vi "UART_Firmware_MultiUp.vi"() -> ()   [LabVIEW 2012]
uses:
  <vilib>/Platform/TimedLoop/XDataNode/timing_clust.ctl
  <vilib>/Platform/TimedLoop/XDataNode/nitl_modes.ctl
  <vilib>/Platform/TimedLoop/XDataNode/wakeup.ctl
  UART/UART_Command.ctl
  <vilib>/rvi/eio/common/nirviEmuTemplateMethod_errors.vi
  <vilib>/rvi/Emulation/niFpgaSctlEmulationRegisterWithScheduler.vi
  <vilib>/rvi/Emulation/niFpgaSctlEmulationScheduler.vi
  <vilib>/eio/EIONode/EIONode.xnode
  <vilib>/Platform/TimedLoop/XDataNode/XDataNode.xnode
  UART/UART_Firmware.lvlib
  <vilib>/Platform/TimedLoop/XDataNode/XDNodeRunTimeDep.lvlib
panel:
  out "FPGA Initialization Complete?":bool
  out "Maximum Nup?":u8
  out "Rx1 FIFO T.O.?":bool
  out "Rx FIFO T.O.?":bool
  out "Tx FIFO T.O.?":bool
  out "Rx0 FIFO T.O.?":bool
  out "IO Module Pre Setup Complete?":bool
  out "Set Voltage Done":bool
  in  "Voltage_Family":u8=4
  out "IO Enabled":bool
  out "DCM_Locked":bool
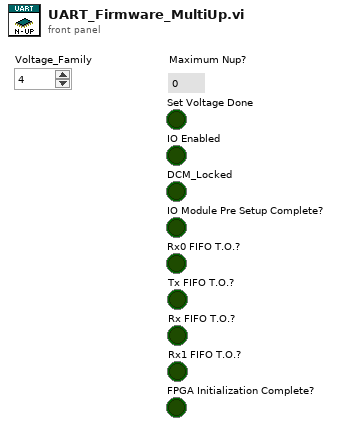
[diagram p1: front panel]
types:
  T1 = typedef "UART_Firmware.lvlib/UART_Command.ctl" = enum8{"None", "Tx", "SetBaud_High", "SetBaud_Low", "SetCharLength", "SetParity", "SetStopBits", "SetSpacing_High", "SetSpacing_Low"}
  T2 = typedef "XDNodeRunTimeDep.lvlib/timing_clust.ctl" = cluster{"Expected End [f-1]":u64, "Actual End [f-1]":u64, "Finished Late? [f-1]":bool, "Expected End [i-1]":u64, "Actual End [i-1]":u64, "Finished Late? [i-1]":bool, "Expected Start [i]":u64, "Actual Start [i]":u64, "Expected Start [f]":u64, "Actual Start [f]":u64, "Source Name":string, "Structure Name":string, "Period":i64, "Deadline":i64, "Offset":i64, "Start":i64, "Priority":i32, "Timeout":i32, "Mode":T3, "Wakeup Reason":T4, "Error":errorcluster, "Source Type":string, "Secondary Source Type":string, "Global End Time":u64, "Global Start Time":u64, "Frame Duration":u64, "Iteration Duration":u64, "Assigned CPU":i32, "I/O Scan Engine Mode":u32}
  T3 = typedef "XDNodeRunTimeDep.lvlib/nitl_modes.ctl" = enum32{"No Change", "Process missed periods, maintain original phase", "Discard missed periods, maintain original phase", "Process missed periods, ignore original phase", "Discard missed periods, ignore original phase"}
  T4 = typedef "XDNodeRunTimeDep.lvlib/wakeup.ctl" = enum32{"Normal", "Aborted", "Asynchronous wakeup", "Timing source error", "Timed loop error", "Timeout"}
  T5 = typedef "UART_Firmware.lvlib/UART_Response.ctl" = enum8{"None", "Rx", "BaudHighAck", "BaudLowAck", "CharSizeAck", "ParityAck", "StopBitsAck", "SpacingHighAck", "SpacingLowAck", "ParityError", "FrameError"}
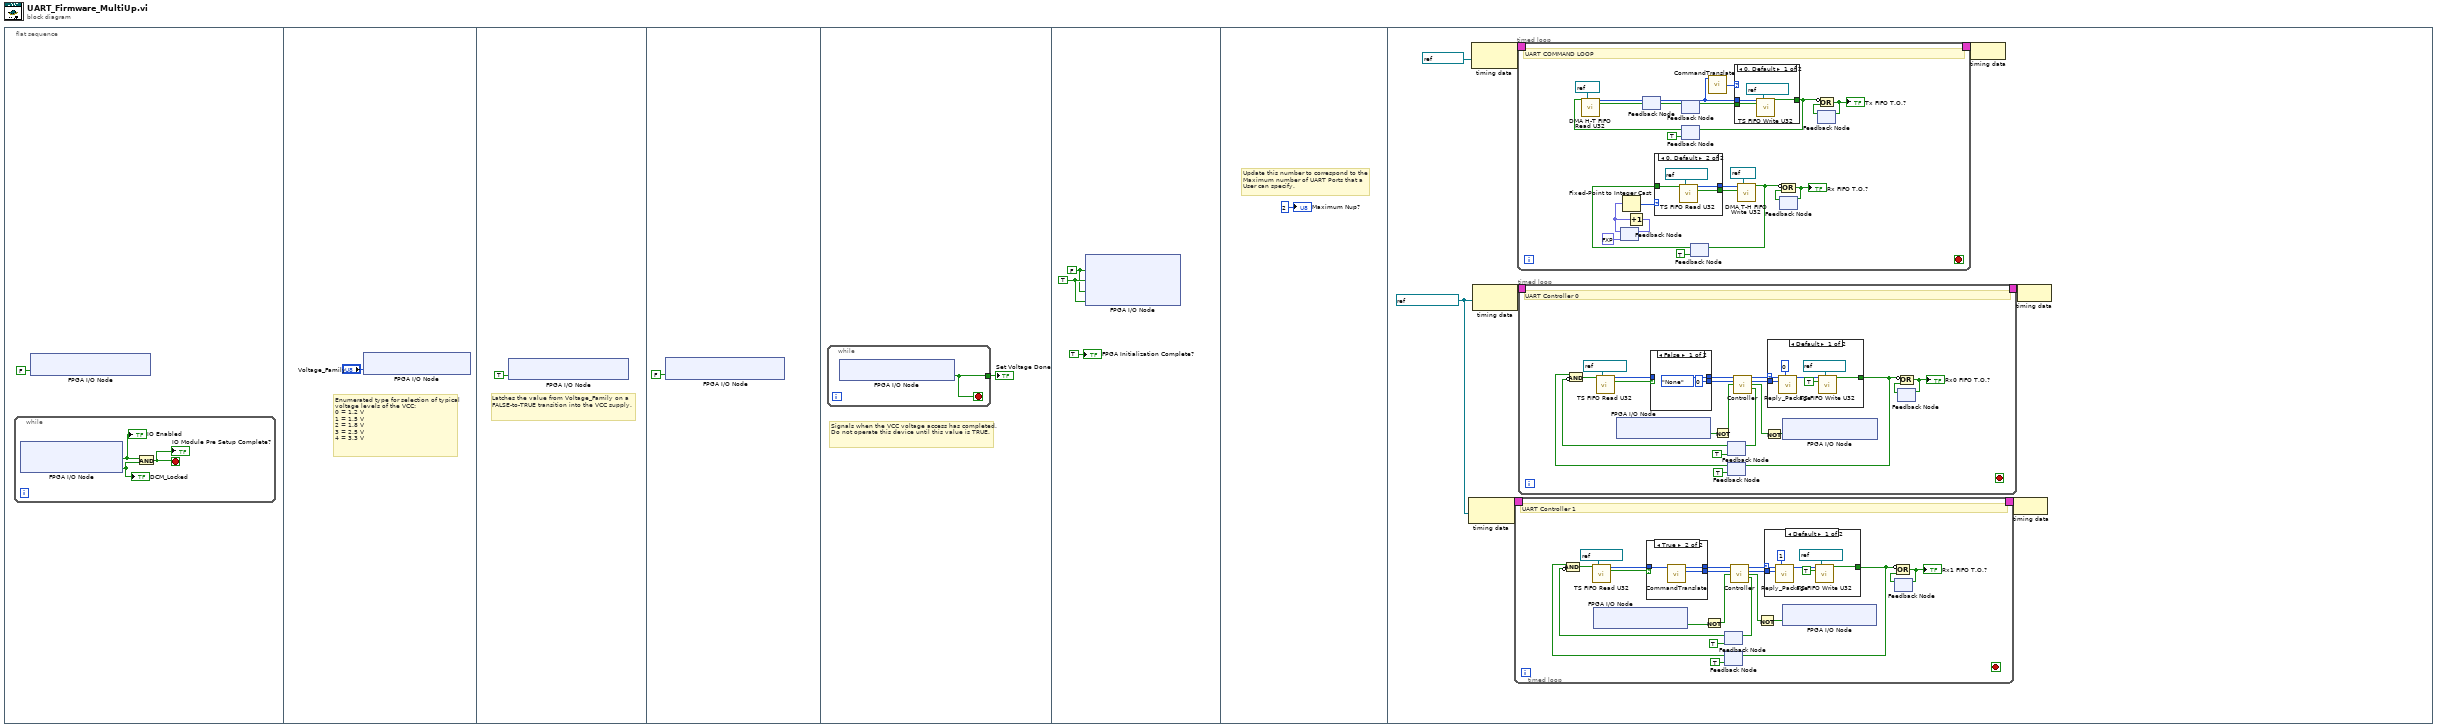
[diagram p0: block diagram]
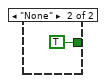
[diagram p2: hidden frame]
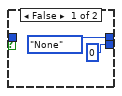
[diagram p3: hidden frame]
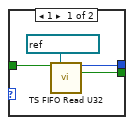
[diagram p4: hidden frame]
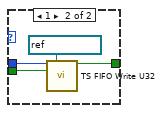
[diagram p5: hidden frame]
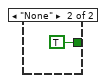
[diagram p6: hidden frame]
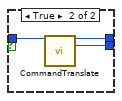
[diagram p7: hidden frame]
diagram:
  n1 = flat-sequence {
    frame #0 {
      n2 = while {
        stop <- w2 stop-if-true
        n3 = xnode "FPGA I/O Node"() -> ("IO Module IO Enabled"=w4:bool, "IO Module\\DCM_Locked"=w3:bool)  [unwired: 2 in, 2 out]
        "IO Enabled" <- w4
        "DCM_Locked" <- w3
        n4 = And(x=w4, y=w3) -> (x .and. y?=w2:bool)
        "IO Module Pre Setup Complete?" <- w2
      }
      n5 = xnode "FPGA I/O Node"("IO Module\\Set_Voltage_Family"=FALSE ("IO Module\\Set_Voltage_Family")) -> ()  [unwired: 1 in, 1 out]
    }
    frame #1 {
      # "Enumerated type for selection of typical\nvoltage levels of the VCC:\n0 = 1.2 V\n1 = 1.5 V\n2 = 1.8 V\n3 = 2.5 V\n4 = 3.3 V"
      n6 = xnode "FPGA I/O Node"("IO Module\\Voltage_Family"="Voltage_Family") -> ()  [unwired: 1 in, 1 out]
    }
    frame #2 {
      # "Latches the value from Voltage_Family on a\nFALSE-to-TRUE transition into the VCC supply."
      n7 = xnode "FPGA I/O Node"("IO Module\\Set_Voltage_Family"=TRUE ("IO Module\\Set_Voltage_Family")) -> ()  [unwired: 1 in, 1 out]
    }
    frame #3 {
      n8 = xnode "FPGA I/O Node"("IO Module\\Set_Voltage_Family"=FALSE ("IO Module\\Set_Voltage_Family")) -> ()  [unwired: 1 in, 1 out]
    }
    frame #4 {
      # "Signals when the VCC voltage access has completed.\nDo not operate this device until this value is TRUE."
      n9 = while {
        tunnel: [w9] -> w8
        stop <- w9 stop-if-true
        n10 = xnode "FPGA I/O Node"() -> ("IO Module\\Set_Voltage_Done"=w9:bool)  [unwired: 1 in, 1 out]
      }
      "Set Voltage Done" <- w8
    }
    frame #5 {
      w11 = TRUE ("IO Module\\SE_Ch1_Dir")
      w10 = FALSE ("IO Module\\SE_Ch0_Dir")
      n11 = xnode "FPGA I/O Node"("IO Module\\SE_PFI1_Dir"=w10, "IO Module\\SE_PFI2_Dir"=w11, "IO Module\\SE_Ch2_Dir"=w10, "IO Module\\SE_Ch3_Dir"=w11) -> ()  [unwired: 4 in, 4 out]
      "FPGA Initialization Complete?" <- TRUE
    }
    frame #6 {
      # "Update this number to correspond to the\nMaximum number of UART Ports that a\nUser can specify."
      "Maximum Nup?" <- u8 2 ("Maximum Nup?")
    }
    frame #7 {
      w14 = refnum<k21> "100 MHz Clock" ("FPGA Clock")
      n12 = node-c288(w14) -> (w16:T2)
      n13 = node-c288(refnum<k21> "105MHz" ("Source Name")) -> (w19:T2)
      n14 = node-c288(w14) -> (w21:T2)
      n15 = timed-loop {
        timing: w16 -> [_]
        timing-out: [_] -> w15
        stop <- _ stop-if-true
        # "UART Controller 1"
        n16 = xnode "FPGA I/O Node"() -> ("IO Module\\SE_Ch2_Rd"=w23:bool)  [unwired: 1 in, 1 out]
        n17 = Not(x=w23) -> (.not. x?=w30:bool)
        n18 = feedback #1(TRUE ("TX_Busy")) -> (w26:bool)
        n19 = feedback #2(TRUE ("Ready for Input?")) -> (w25:bool)
        n20 = Compound Arithmetic op=AND(w25, invert w26) -> (w33:bool)
        n21 = call "TS FIFO Read U32.vi"("Ready for Output?"=w33, "FIFO In"=refnum<k21> "Tx_Port1") -> ("Data Out"=w37:u32, "Data Valid?"=w38:bool)  [unwired: 12 in]
        n22 = case shown="True" w38 {
          tunnel: [UART_Command."None" ("UART_Command") w53] -> w32
          tunnel: [u16 0 ("Cmd_data") w52] -> w31
          tunnel: w37 -> [_ w54]
          frame False {
          }
          frame True {
            n23 = call "CommandTranslate.vi"("raw_command"=w54) -> ("UART_Command"=w53:T1, "Cmd_data"=w52:u16)  [unwired: 12 in, 1 out]
          }
        }
        n24 = call "Controller.vi"("UART_Command"=w32, "Cmd_data"=w31, "RX"=w30) -> ("UART_Reply"=w29:T5, "Reply_data"=w28:u16, "TX"=w27:bool, "TX_Busy"=w24:bool)  [unwired: 7 in, 2 out]
        n25 = feedback-in #1(w24) -> ()
        n26 = Not(x=w27) -> (.not. x?=w22:bool)
        n27 = case shown="Default" w29 {
          selector: w29 -> [w45 _]
          tunnel: [w46 TRUE ("Ready for Input?")] -> w35
          tunnel: w28 -> [w42 _]
          frame Default {
            n28 = call "Reply_Package.vi"("UART Reply"=w45, "UART_Ch"=u8 1, "Reply Data"=w42) -> ("Reply packed"=w44:u32)  [unwired: 12 in]
            n29 = call "TS FIFO Write U32.vi"("Data In"=w44, "FIFO In"=refnum<k21> "Rx_Port1", "Input Valid"=TRUE) -> ("Ready for Input?"=w46:bool)  [unwired: 12 in]
          }
          frame "None" {
          }
        }
        n30 = feedback-in #2(w35) -> ()
        n31 = xnode "FPGA I/O Node"("IO Module\\SE_Ch3_Wr"=w22) -> ()  [unwired: 1 in, 1 out]
        n32 = feedback #3() -> (w39:bool)  [unwired: 1 in]
        n33 = Compound Arithmetic op=OR(invert w35, w39) -> (w40:bool)
        "Rx1 FIFO T.O.?" <- w40
        n34 = feedback-in #3(w40) -> ()
      }
      n35 = timed-loop {
        timing: w19 -> [_]
        timing-out: [_] -> w18
        stop <- _ stop-if-true
        # "UART COMMAND LOOP"
        n36 = feedback #4(fxp<+,1,1> 0.0) -> (w71:fxp<+,1,1>)
        n37 = Fixed-Point to Integer Cast(1:w71) -> (0:w69:u8)
        n38 = Increment(x=w71) -> (x+1=w70:fxp<+,1,1>)
        n39 = feedback-in #4(w70) -> ()
        n40 = feedback #5() -> (w61:u32)  [unwired: 1 in]
        n41 = feedback #6(TRUE ("Ready for Input?")) -> (w80:bool)
        n42 = call "DMA H-T FIFO Read U32.vi"("Ready for Output?"=w80, "FIFO In"=refnum<k21> "TX") -> ("Data Out"=w81:u32, "Data Valid?"=w82:bool)  [unwired: 12 in]
        n43 = feedback-in #5(w81) -> ()
        n44 = feedback-in #7(w82) -> ()
        n45 = feedback #7() -> (w78:bool)  [unwired: 1 in]
        n46 = feedback #8(TRUE ("Ready for Input?")) -> (w68:bool)
        n47 = case shown="0, Default" w69 {
          tunnel: [w86 w90] -> w74
          tunnel: [w85 w89] -> w75
          tunnel: w68 -> [w84 w88]
          frame 1 {
            n48 = call "TS FIFO Read U32.vi"("Ready for Output?"=w84, "FIFO In"=refnum<k21> "Rx_Port1") -> ("Data Out"=w85:u32, "Data Valid?"=w86:bool)  [unwired: 12 in]
          }
          frame 0, Default {
            n49 = call "TS FIFO Read U32.vi"("Ready for Output?"=w88, "FIFO In"=refnum<k21> "Rx_Port0") -> ("Data Out"=w89:u32, "Data Valid?"=w90:bool)  [unwired: 12 in]
          }
        }
        n50 = call "CommandTranslate.vi"("raw_command"=w61) -> ("UART_Ch"=w62:u8)  [unwired: 12 in, 2 out]
        n51 = case shown="0, Default" w62 {
          tunnel: w78 -> [w94 w98]
          tunnel: [w93 w97] -> w66
          tunnel: w61 -> [w92 w96]
          frame 0, Default {
            n52 = call "TS FIFO Write U32.vi"("Data In"=w92, "FIFO In"=refnum<k21> "Tx_Port0", "Input Valid"=w94) -> ("Ready for Input?"=w93:bool)  [unwired: 12 in]
          }
          frame 1 {
            n53 = call "TS FIFO Write U32.vi"("Data In"=w96, "FIFO In"=refnum<k21> "Tx_Port1", "Input Valid"=w98) -> ("Ready for Input?"=w97:bool)  [unwired: 12 in]
          }
        }
        n54 = feedback-in #6(w66) -> ()
        n55 = call "DMA T-H FIFO Write U32.vi"("Data In"=w75, "FIFO In"=refnum<k21> "RX", "Input Valid"=w74) -> ("Ready for Input?"=w63:bool)  [unwired: 12 in]
        n56 = feedback-in #8(w63) -> ()
        n57 = feedback #9() -> (w64:bool)  [unwired: 1 in]
        n58 = Compound Arithmetic op=OR(invert w63, w64) -> (w65:bool)
        "Rx FIFO T.O.?" <- w65
        n59 = feedback-in #9(w65) -> ()
        n60 = feedback #10() -> (w77:bool)  [unwired: 1 in]
        n61 = Compound Arithmetic op=OR(invert w66, w77) -> (w76:bool)
        "Tx FIFO T.O.?" <- w76
        n62 = feedback-in #10(w76) -> ()
      }
      n63 = timed-loop {
        timing: w21 -> [_]
        timing-out: [_] -> w20
        stop <- _ stop-if-true
        # "UART Controller 0"
        n64 = xnode "FPGA I/O Node"() -> ("IO Module\\SE_PFI1_Rd"=w109:bool)  [unwired: 1 in, 1 out]
        n65 = Not(x=w109) -> (.not. x?=w107:bool)
        n66 = feedback #11(TRUE ("TX_Busy")) -> (w112:bool)
        n67 = feedback #12(TRUE ("Ready for Input?")) -> (w111:bool)
        n68 = Compound Arithmetic op=AND(w111, invert w112) -> (w117:bool)
        n69 = call "TS FIFO Read U32.vi"("Ready for Output?"=w117, "FIFO In"=refnum<k21> "Tx_Port0") -> ("Data Out"=w121:u32, "Data Valid?"=w122:bool)  [unwired: 12 in]
        n70 = case shown="False" w122 {
          tunnel: [UART_Command."None" ("UART_Command") w137] -> w116
          tunnel: [u16 0 ("Cmd_data") w136] -> w115
          tunnel: w121 -> [_ w138]
          frame False {
          }
          frame True {
            n71 = call "CommandTranslate.vi"("raw_command"=w138) -> ("UART_Command"=w137:T1, "Cmd_data"=w136:u16)  [unwired: 12 in, 1 out]
          }
        }
        n72 = call "Controller.vi"("UART_Command"=w116, "Cmd_data"=w115, "RX"=w107) -> ("UART_Reply"=w114:T5, "Reply_data"=w113:u16, "TX"=w108:bool, "TX_Busy"=w110:bool)  [unwired: 7 in, 2 out]
        n73 = feedback-in #11(w110) -> ()
        n74 = Not(x=w108) -> (.not. x?=w106:bool)
        n75 = case shown="Default" w114 {
          selector: w114 -> [w129 _]
          tunnel: [w130 TRUE ("Ready for Input?")] -> w119
          tunnel: w113 -> [w126 _]
          frame Default {
            n76 = call "Reply_Package.vi"("UART Reply"=w129, "UART_Ch"=u8 0, "Reply Data"=w126) -> ("Reply packed"=w128:u32)  [unwired: 12 in]
            n77 = call "TS FIFO Write U32.vi"("Data In"=w128, "FIFO In"=refnum<k21> "Rx_Port0", "Input Valid"=TRUE) -> ("Ready for Input?"=w130:bool)  [unwired: 12 in]
          }
          frame "None" {
          }
        }
        n78 = feedback-in #12(w119) -> ()
        n79 = xnode "FPGA I/O Node"("IO Module\\SE_PFI2_Wr"=w106) -> ()  [unwired: 1 in, 1 out]
        n80 = feedback #13() -> (w123:bool)  [unwired: 1 in]
        n81 = Compound Arithmetic op=OR(invert w119, w123) -> (w124:bool)
        "Rx0 FIFO T.O.?" <- w124
        n82 = feedback-in #13(w124) -> ()
      }
      n83 = node-c288(w18) -> ()
      n84 = node-c288(w15) -> ()
      n85 = node-c288(w20) -> ()
    }
  }
